vi "Results_file_header.vi"() -> (0 "Header":string)   [LabVIEW 2017]
uses:
  Controls/Post_Process.ctl
  Globals/Meas_global.vi
panel:
  # "Create file Header"
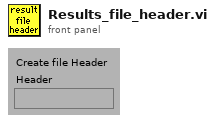
[diagram p1: front panel]
types:
  T1 = typedef "Post_Process.ctl" = enum16{"Take New Data", "Post Process Raw Data File"}
  T2 = typedef "Ch_and_Spans.ctl" = cluster{"Sync Delay (ms)":dbl, "Ch No":i16, "Var name":string, "Use Latest Calib":bool}
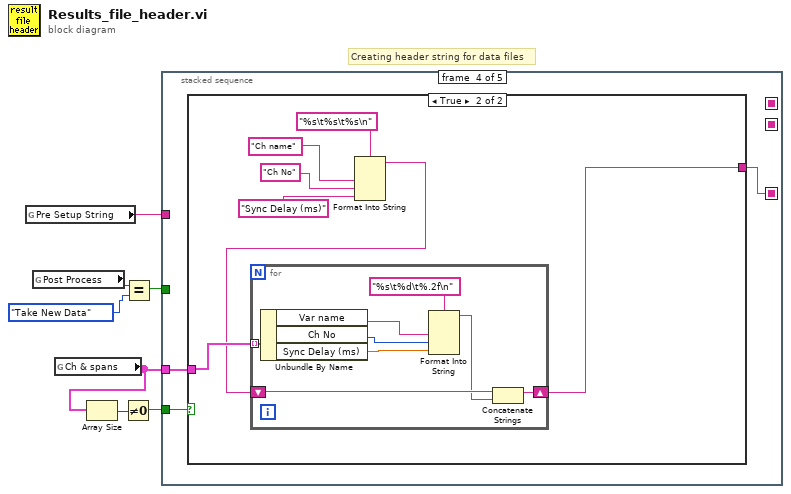
[diagram p0: block diagram]
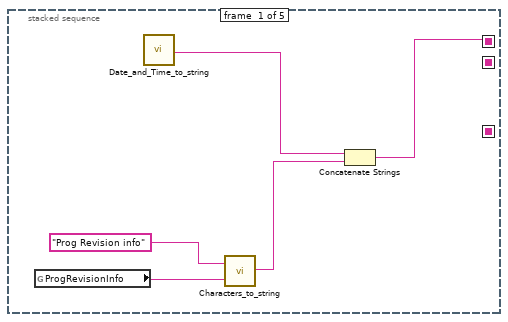
[diagram p2: hidden frame]
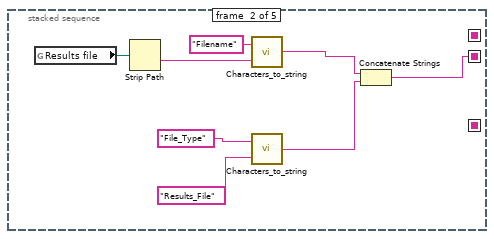
[diagram p3: hidden frame]
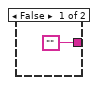
[diagram p5: hidden frame]
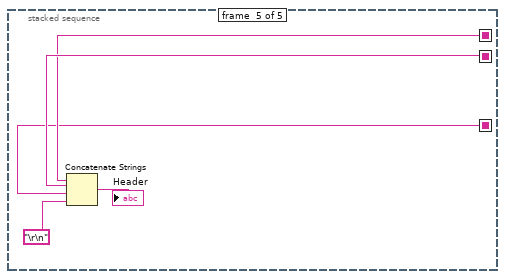
[diagram p6: hidden frame]
diagram:
  # "Creating header string for data files"
  n1 = global read "Meas_global.vi" "Pre Setup String"() -> (w2:string)
  n2 = global read "Meas_global.vi" "Post Process"() -> (w7:T1)
  n3 = global read "Meas_global.vi" "Ch & spans"() -> (w4:T2[])
  n4 = Array Size(array=w4) -> (size(s)=w5:i32)
  n5 = Not Equal To 0?(x=w5) -> (x != 0?=w3:bool)
  n6 = Equal?(x=w7, y=Post_Process."Take New Data" ("Post Process")) -> (x = y?=w6:bool)
  n7 = stacked-sequence {
    seq-local: [_ w13 _ _ _] -> [_ _ _ _ w44]
    seq-local: [w9 _ _ _ _] -> [_ _ _ _ w42]
    seq-local: [_ _ _ w21 _] -> [_ _ _ _ w41]
    tunnel: w6 -> [_ _ _ _ _]
    tunnel: w4 -> [_ _ _ w22 _]
    tunnel: w3 -> [_ _ _ w23 _]
    tunnel: w2 -> [_ _ _ _ _]
    frame #0 {
      n8 = global read "Meas_global.vi" "ProgRevisionInfo"() -> (w8:string)
      n9 = call "Date_and_Time_to_string.vi"() -> ("Date and time (spreadsheet)"=w10:string)
      n10 = call "Characters_to_string.vi"("Characters to write"=w8, "Label for characters"="Prog Revision info") -> ("Output string"=w11:string)
      n11 = Concatenate Strings(w10, w11) -> (w9:string)
    }
    frame #1 {
      n12 = global read "Meas_global.vi" "Results file"() -> (w19:path)
      n13 = Strip Path(path=w19) -> (name=w18:string)  [unwired: 1 out]
      n14 = call "Characters_to_string.vi"("Characters to write"=w18, "Label for characters"="Filename") -> ("Output string"=w15:string)
      n15 = call "Characters_to_string.vi"("Characters to write"="Results_File", "Label for characters"="File_Type") -> ("Output string"=w14:string)
      n16 = Concatenate Strings(w15, w14) -> (w13:string)
    }
    frame #2 {
    }
    frame #3 {
      n17 = case shown="True" w23 {
        tunnel: w22 -> [_ w27]
        tunnel: ["" w25] -> w21
        frame False {
        }
        frame True {
          n18 = Format Into String(format string="%s\t%s\t%s\n" ("Format String"), "Ch name", "Ch No", "Sync Delay (ms)") -> (resulting string=w26:string)  [unwired: 2 in, 1 out]
          n19 = for {
            tunnel: w27 -> [w39] mode=indexing
            shift-right: [w32] -> w25
            shift-left: w26 -> [w34]
            n20 = Unbundle By Name(w39) -> ("Var name"=w38:string, "Ch No"=w37:i16, "Sync Delay (ms)"=w36:dbl)
            n21 = Format Into String(format string="%s\t%d\t%.2f\n" ("Format String"), w38, w37, w36) -> (resulting string=w33:string)  [unwired: 2 in, 1 out]
            n22 = Concatenate Strings(w34, w33) -> (w32:string)
          }
        }
      }
    }
    frame #4 {
      n23 = Concatenate Strings(w42, w44, w41, "\r\n") -> (→"Header":string)
    }
  }
